vi "Set Device Parameters.vi"(8 "error in":errorcluster, 10 "device parameters":T1, 11 "Ballard ARINC 429 custom device in":T3=18446744073709551615 format="%.0x") -> (0 "error out":errorcluster, 3 "Ballard ARINC 429 custom device out":T3 format="%.0x")   [LabVIEW 2020, in "Ballard ARINC 429 Scripting.lvlib"]
uses:
  <vilib>/addons/VeriStand Custom Device Scripting APIs/Ballard ARINC 429/Custom Device Support/Scripting/Ballard/Ballard ARINC 429 Scripting.lvlib
  <vilib>/NI VeriStand/Custom Device API/Custom Device Item Ref.ctl
  <vilib>/addons/VeriStand Custom Device Scripting APIs/Ballard ARINC 429/Custom Device Support/Shared/Device Parameters.ctl
  <vilib>/addons/VeriStand Custom Device Scripting APIs/Ballard ARINC 429/Custom Device Support/Shared/Initialization Method.ctl
  <vilib>/addons/VeriStand Custom Device Scripting APIs/Ballard ARINC 429/Custom Device Support/Scripting/Ballard/Constants.vi
  <vilib>/NI VeriStand/Custom Device API/Set Item Property (U16).vi
  <vilib>/NI VeriStand/Custom Device API/Set Item Property (I32).vi
  <vilib>/NI VeriStand/Custom Device API/Custom Device API.lvlib
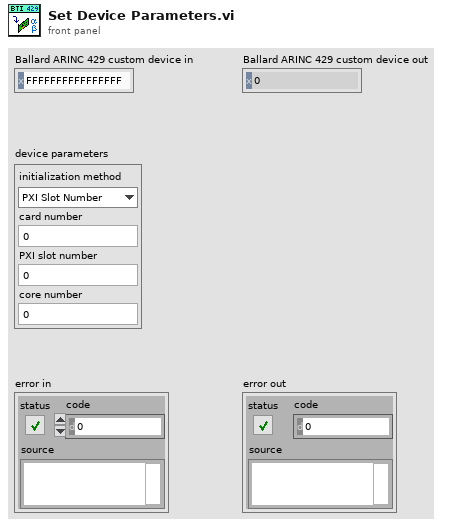
[diagram p1: front panel]
types:
  T1 = typedef "Device Parameters.ctl" = cluster{"initialization method":T2, "card number":i32, "PXI slot number":i32, "core number":i32}
  T2 = typedef "Initialization Method.ctl" = enum16{"PXI Slot Number", "Card Number"}
  T3 = typedef "Custom Device API.lvlib/Custom Device Item Ref.ctl" = u64
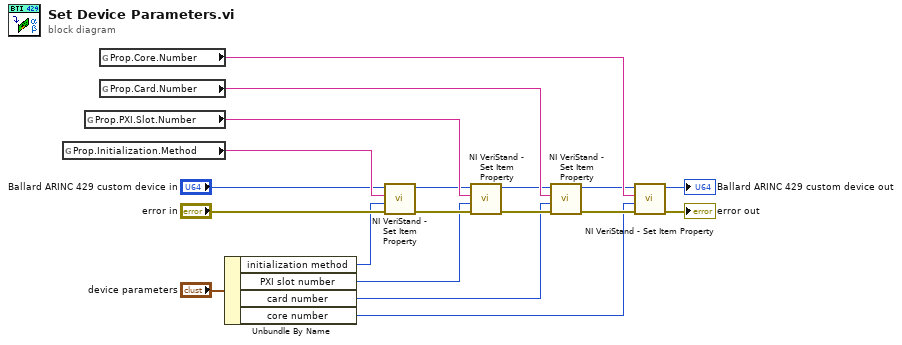
[diagram p0: block diagram]
diagram:
  n1 = global read "Constants.vi" "Prop.Initialization.Method"() -> (w16:string)
  n2 = global read "Constants.vi" "Prop.PXI.Slot.Number"() -> (w19:string)
  n3 = global read "Constants.vi" "Prop.Core.Number"() -> (w17:string)
  n4 = global read "Constants.vi" "Prop.Card.Number"() -> (w18:string)
  n5 = Unbundle By Name("device parameters") -> ("initialization method"=w4:T2, "PXI slot number"=w3:i32, "card number"=w2:i32, "core number"=w1:i32)
  n6 = call-poly <vilib>:"NI VeriStand - Set Item Property.vi"("error in (no error)"="error in", "Value"=w4, "Property Name"=w16, "Item Ref in"="Ballard ARINC 429 custom device in") -> ("error out"=w9:errorcluster, "Item Ref out"=w8:T3)  [unwired: 5 in, 1 out]
  n7 = call-poly <vilib>:"NI VeriStand - Set Item Property.vi"("error in (no error)"=w9, "Value"=w3, "Property Name"=w19, "Item Ref in"=w8) -> ("error out"=w14:errorcluster, "Item Ref out"=w15:T3)  [unwired: 5 in, 1 out]
  n8 = call-poly <vilib>:"NI VeriStand - Set Item Property.vi"("error in (no error)"=w14, "Value"=w2, "Property Name"=w18, "Item Ref in"=w15) -> ("error out"=w12:errorcluster, "Item Ref out"=w13:T3)  [unwired: 5 in, 1 out]
  n9 = call-poly <vilib>:"NI VeriStand - Set Item Property.vi"("error in (no error)"=w12, "Value"=w1, "Property Name"=w17, "Item Ref in"=w13) -> ("error out"=→"error out":errorcluster, "Item Ref out"=→"Ballard ARINC 429 custom device out":T3)  [unwired: 5 in, 1 out]
